vi "Create Notifiers.vi"(7 "Notifiers":T1, 11 "error in":errorcluster) -> (0 "error in 2":errorcluster)   [LabVIEW 2015]
uses:
  Notifier.ctl
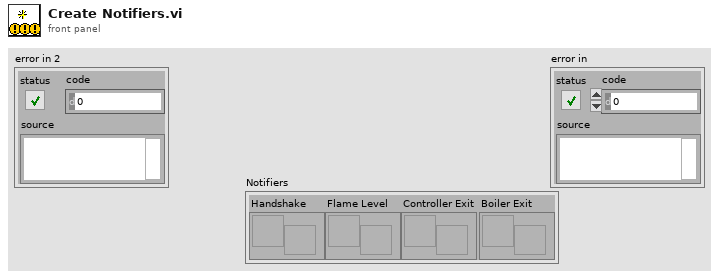
[diagram p1: front panel]
types:
  T1 = typedef "Notifier.ctl" = cluster{"Handshake":refnum<notifier>, "Flame Level":refnum<notifier>, "Controller Exit":refnum<notifier>, "Boiler Exit":refnum<notifier>}
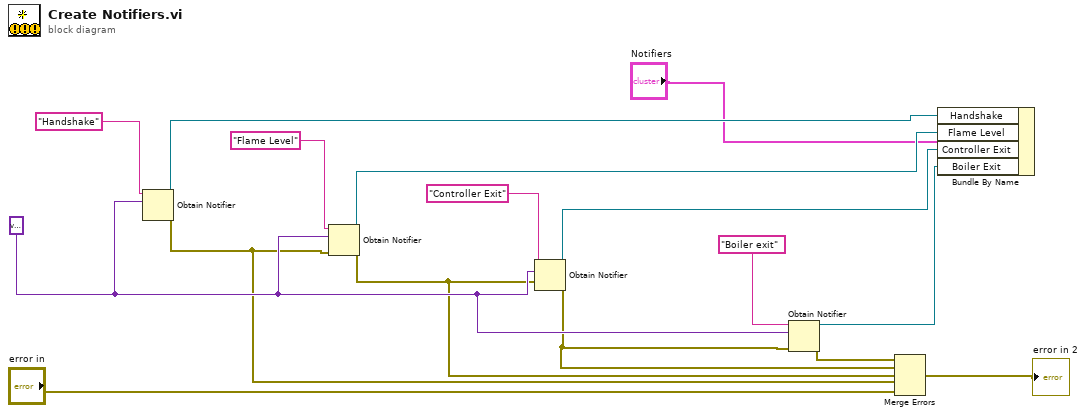
[diagram p0: block diagram]
diagram:
  w14 = variant
  n1 = Obtain Notifier(name (unnamed)="Handshake", notification data type=w14) -> (notifier out=w2:refnum<notifier>, error out=w10:errorcluster)  [unwired: 2 in, 1 out]
  n2 = Obtain Notifier(name (unnamed)="Flame Level", notification data type=w14, error in (no error)=w10) -> (notifier out=w3:refnum<notifier>, error out=w11:errorcluster)  [unwired: 1 in, 1 out]
  n3 = Obtain Notifier(name (unnamed)="Controller Exit", notification data type=w14, error in (no error)=w11) -> (notifier out=w4:refnum<notifier>, error out=w12:errorcluster)  [unwired: 1 in, 1 out]
  n4 = Obtain Notifier(name (unnamed)="Boiler exit", notification data type=w14, error in (no error)=w12) -> (notifier out=w5:refnum<notifier>, error out=w13:errorcluster)  [unwired: 1 in, 1 out]
  n5 = Merge Errors(w13, w12, w11, w10, "error in") -> (→"error in 2":errorcluster)
  n6 = Bundle By Name(cluster="Notifiers", "Handshake"=w2, "Flame Level"=w3, "Controller Exit"=w4, "Boiler Exit"=w5) -> ()  [unwired: 1 out]
